vi "MonitoringProcess_DAQ.vi"(8 "error in (no error)":errorcluster, 9 "start process sync notifier":refnum<notifier>, 10 "TopLevel":refnum<class "TopLevel.lvclass">, 11 "DAQ":refnum<class "DAQ.lvclass">) -> (0 "error out":errorcluster)   [LabVIEW 2022 SP3, in "DAQ.lvclass"]
doc: "Developed by Kevin Thompson\nkevin@thompsonengineering.net\n\nCopyright 2015\nThompson Engineering, LLC"
uses:
  DAQ.lvclass
  TopLevel/TopLevel.lvclass
  MonitorProcess_DAQ SM AppData--cluster.ctl
  DataTypes/TD DAQ Settings--cluster.ctl
  DataTypes/TD DI Instrument Settings--cluster.ctl
  DataTypes/TD AI Instrument Settings--cluster.ctl
  DataTypes/TD AI InstSettings--cluster.ctl
  ProcessSupport/TD SimAI Ranges--cluster.ctl
  DAQ_Common/DataTypes/Timer_Data--Cluster.ctl
  <vilib>/TELLC/Dynamic CVT API/TD Dynamic CVT DVR--ref.ctl
  DAQ.lvclass/DAQ.ctl
  TopLevel/Typedefs/PrimingMode APIData.ctl
  TopLevel/Typedefs/PurgeMode--Enum.ctl
  TopLevel/Typedefs/PrinterHeads--Enum.ctl
  IO/Typedefs/ICP2-DO Channel Names.ctl
  DataTypes/TD DAQ Output EventSenderMode-enum.ctl
  Accessors/Get DAQ Settings.vi
  TopLevel/PurgeRequestWindow--Process.vi
  DAQ_Common/Lib/ErrorHandler/ErrorHandler.lvclass
  IO/IO.lvclass
panel:
  out "SWLED 2":bool
  out "SW LED DO":string
  out "found":bool
  out "SWLED":bool
  out "DIName":string
  in  "injected error cluster":errorcluster
  in  "inject error":bool
  in  "Stop Process":bool
  # "Simulated error injection\nfor testing and debug"
  # "This is for debugging. Process should stop from user event."
  # "Makes sure to set this value from the process caller. Using the Start asyncronous call function."
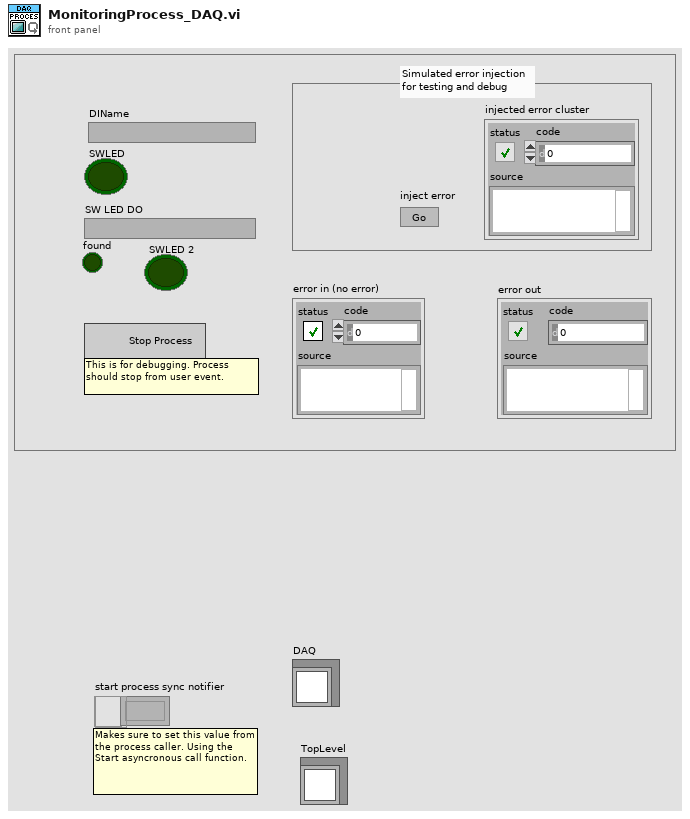
[diagram p1: front panel]
types:
  T1 = typedef "DAQ.lvclass/MonitorProcess_DAQ SM AppData--cluster.ctl" = cluster{"Core":cluster{"Current VI Ref":refnum<vi>, "process sync notifier":refnum<notifier>}, "AsyncSMQ":refnum<queue>, "DAQ Settings":T2, "SimDaqLoopIntv":i32, "ThreadSyncRndzv":T7, "vData":variant, "quitting":bool, "Self Reference":refnum<class "DAQ.lvclass">, "TopLevel":refnum<class "TopLevel.lvclass">, "Timer":T8, "DAQData Dict":T9}
  T2 = typedef "DAQ.lvclass/TD DAQ Settings--cluster.ctl" = cluster{"Simulate DAQ":bool, "DI Settings":T3[], "AI Settings":T4[], "Relay IONames":string[], "AO IONames":string[], "AO NChan SingleTask":bool}
  T3 = typedef "DAQ.lvclass/TD DI Instrument Settings--cluster.ctl" = cluster{"Disable":bool, "DI TaskName":string, "DI RefreshIntv":i32}
  T4 = typedef "DAQ.lvclass/TD AI Instrument Settings--cluster.ctl" = cluster{"Disable":bool, "AI TaskName":string, "AI InstSettings":T5, "SimAI Ranges":T6}
  T5 = typedef "DAQ.lvclass/TD AI InstSettings--cluster.ctl" = cluster{"DaqRate":dbl, "NumSamples":i32}
  T6 = typedef "DAQ.lvclass/TD SimAI Ranges--cluster.ctl" = cluster{"lo":dbl, "hi":dbl}
  T7 = typedef "Rendezvous RefNum" = refnum<k1>
  T8 = typedef "Timer_Data--Cluster.ctl" = cluster{"StartTime":timestamp, "TimerValue":dbl, "Enable":bool, "Expired":bool}
  T9 = typedef "TD Dynamic CVT DVR--ref.ctl" = refnum<data-value>
  T10 = typedef "PurgeMode--Enum.ctl" = enum16{"Pre-Purge", "Purge", "Spit", "Shake"}
  T11 = typedef "TopLevel.lvclass/PrimingMode APIData.ctl" = cluster{"Interval (s)":dbl, "PurgeDuration (s)":dbl, "Repeats":u8, "PrimingMode":T10, "Head":T12, "Frequency (Hz)":i32, "PrintWeight":dbl}
  T12 = typedef "PrinterHeads--Enum.ctl" = enum16{"-1", "1", "2", "3", "4", "5", "6"}
  T13 = typedef "DAQ.lvclass/TD DAQ Output EventSenderMode-enum.ctl" = enum16{"manual", "automation"}
  T14 = typedef "IO.lvclass/ICP2-DO Channel Names.ctl" = enum16{"None", "Meniscus Valve Open - R1", "Meniscus Valve Open - R2", "Meniscus Valve Open - R3", "Meniscus Valve Open - R4", "Meniscus Valve Open - R5", "Meniscus Valve Open - R6", "Ink Flow Valve Open - R1", "Ink Flow Valve Open - R2", "Ink Flow Valve Open - R3", "Ink Flow Valve Open - R4", "Ink Flow Valve Open - R5", "Ink Flow Valve Open - R6", "SW_LED - Ink Valve - R1", "SW_LED - Ink Valve - R2", "SW_LED - Ink Valve - R3", "Recirc Pump On - R1", "Recirc Pump On - R2", "Recirc Pump On - R3", "Recirc Pump On - R4", "Recirc Pump On - R5", "Recirc Pump On - R6", "SW_LED - Ink Valve - R4", "SW_LED - Ink Valve - R5", "SW_LED - Ink Valve - R6"}
  T15 = enum32{"Invalid", "Standard", "Closed", "Hidden", "Minimized", "Maximized"}
  T16 = cluster{"Prime 1":string, "Prime 2":string, "Prime 3":string, "Prime 4":string, "Prime 5":string, "Prime 6":string}
  T17 = typedef "processMode--enum.ctl" = enum16{"Short Idle", "Long Idle ", "C30_Process", "S30_Process"}
  T18 = typedef "ProcessMode--Cluster.ctl" = cluster{"Head Array":u8[], "Head Enable":bool[], "HeadTemp[]":dbl[], "MeniscusPress[]":dbl[], "Recirc[]":bool[], "ProcessModeEnum":T17, "ProcessModeStr":string, "ColorPlane[]":string[]}
  T19 = typedef "TopLevel.lvclass/UserEvents.ctl" = cluster{"API Incoming Event":refnum<user-event>, "API Executed Event":refnum<user-event>, "API Return Event":refnum<user-event>, "Exit Event":refnum<user-event>, "StatusChanged":refnum<user-event>, "DLP GUI Config Changed":refnum<user-event>, "AppEvent":refnum<user-event>, "Login Event":refnum<user-event>, "HeadPrimeStatusEvent":refnum<user-event>}
  T20 = typedef "DAQ.lvclass/TD PublicEvents--cluster.ctl" = cluster{"DaqOutputCmd Ev":refnum<user-event>, "stop process":refnum<user-event>, "DAQ.AsyncCmd Event":refnum<user-event>, "DAQStateChanged Event":refnum<user-event>, "DAQ.AsyncMsg Event":refnum<user-event>, "DAQ_DO_StatusEvent":refnum<user-event>, "DIStateChangeEv":refnum<user-event>, "UI StateChanged":refnum<user-event>, "PurgeTimerEvent":refnum<user-event>}
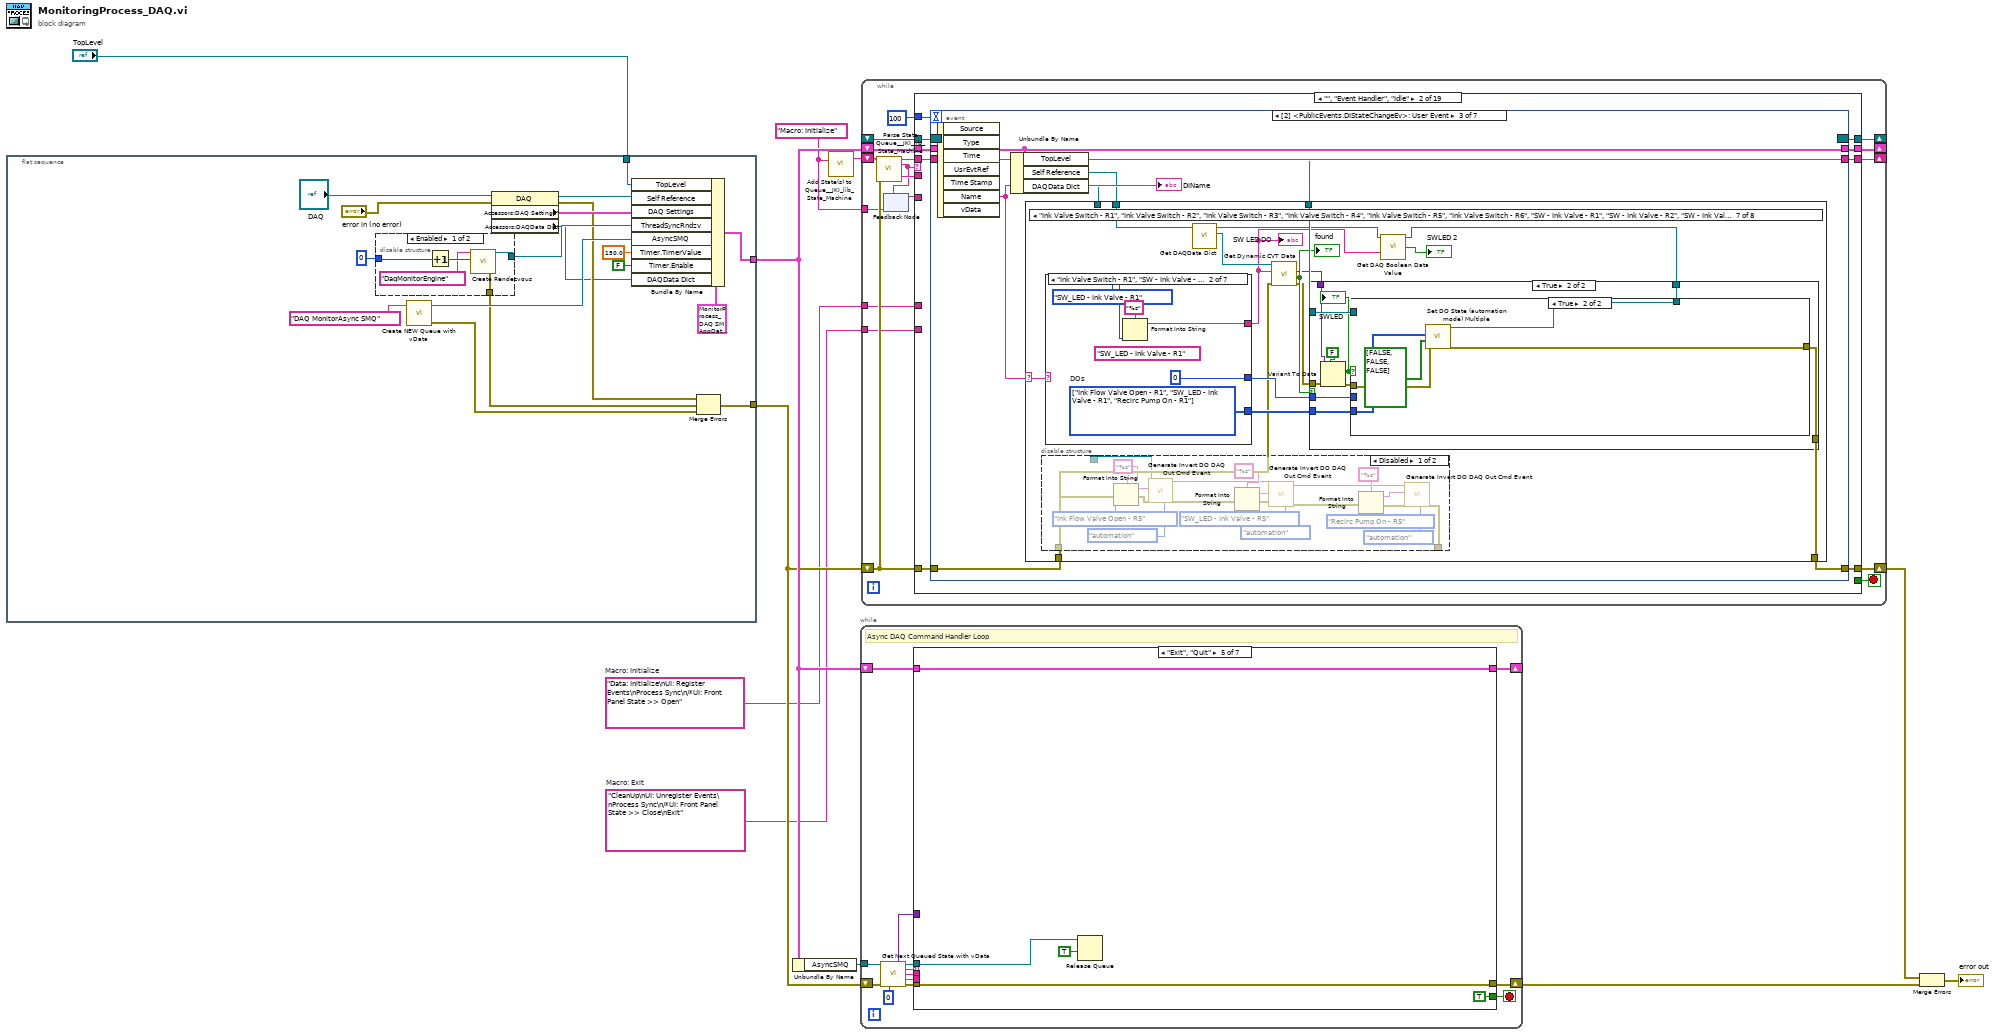
[diagram p0: block diagram]
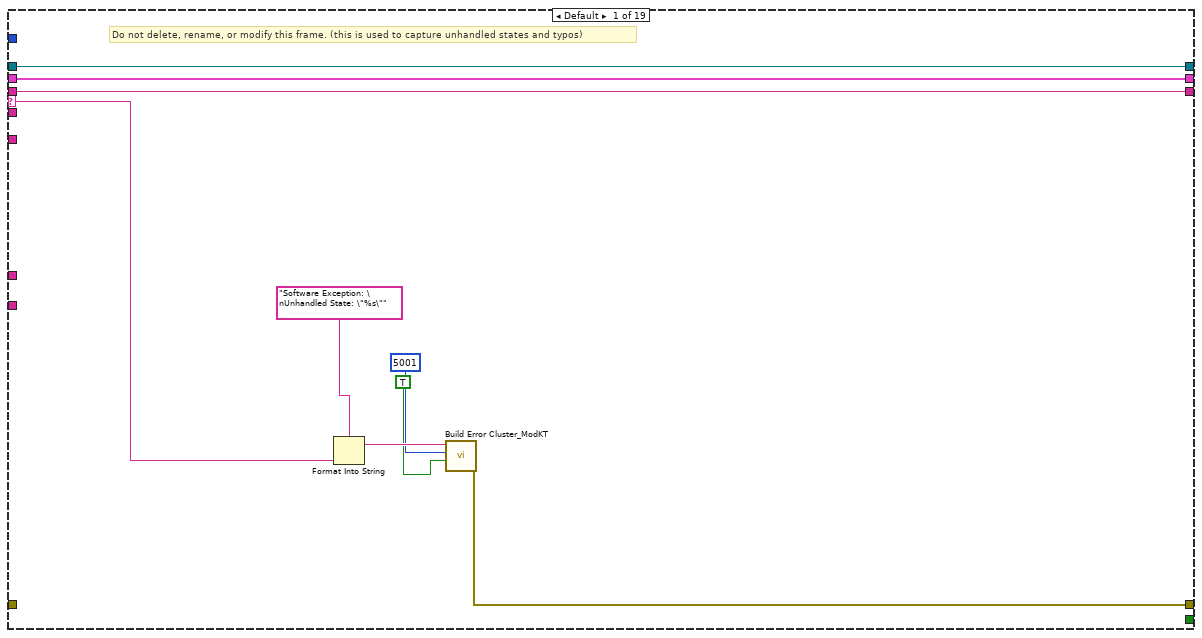
[diagram p2: hidden frame]
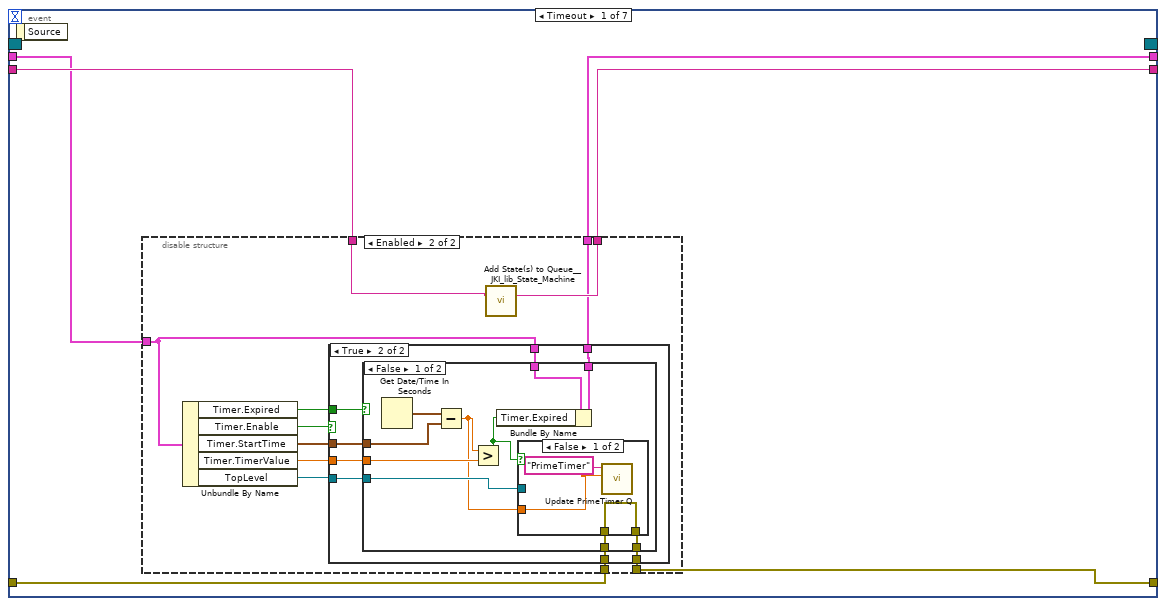
[diagram p3: hidden frame]
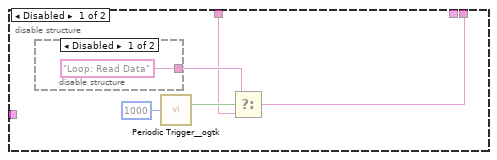
[diagram p4: hidden frame]
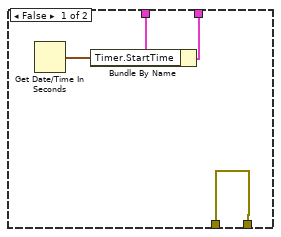
[diagram p6: hidden frame]
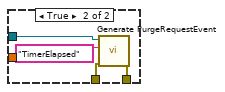
[diagram p7: hidden frame]
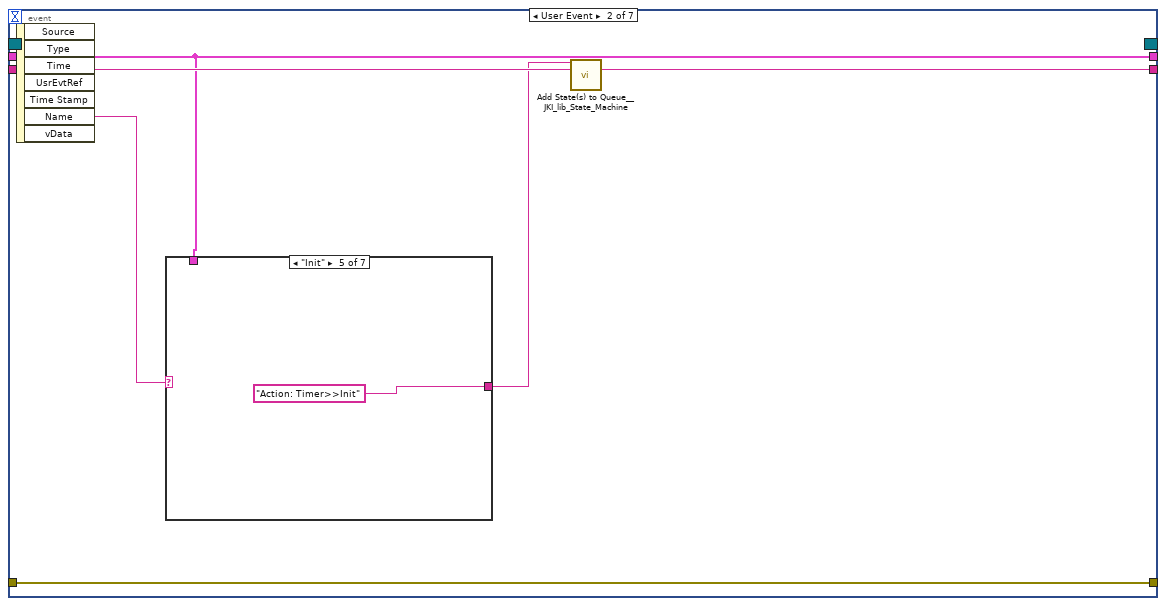
[diagram p9: hidden frame]
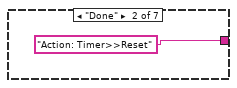
[diagram p11: hidden frame]
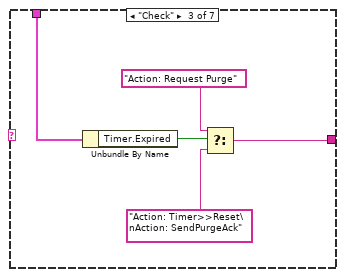
[diagram p12: hidden frame]
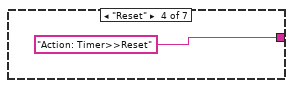
[diagram p13: hidden frame]
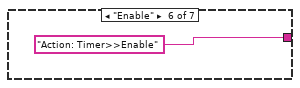
[diagram p14: hidden frame]
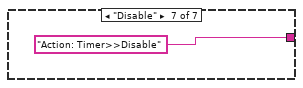
[diagram p15: hidden frame]
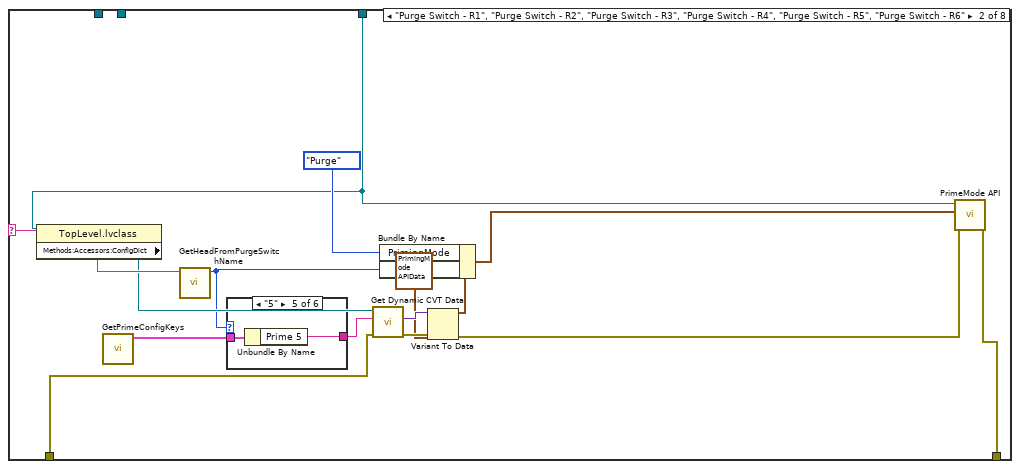
[diagram p17: hidden frame]
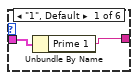
[diagram p18: hidden frame]
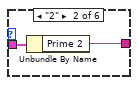
[diagram p19: hidden frame]
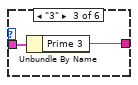
[diagram p20: hidden frame]
diagram:
  w4 = "Data: Initialize\nUI: Register Events\nProcess Sync\n/*UI: Front Panel State >> Open"  # Macro: Initialize
  w3 = "CleanUp\nUI: Unregister Events\nProcess Sync\n/*UI: Front Panel State >> Close\nExit"  # Macro: Exit
  w2 = "Macro: Initialize"
  n1 = flat-sequence {
    tunnel: [w29] -> w9
    tunnel: [w23] -> w8
    tunnel: "TopLevel" -> [w15]
    frame #0 {
      n2 = disable-structure shown="Enabled" {
        disable-tunnel: [w34 _] -> w25
        disable-tunnel: [w33 _] -> w24
        disable-tunnel: 0 -> [w30 _]
        frame Enabled {
          n3 = Increment(x=w30) -> (x+1=w32:i32)
          n4 = call <vilib>:"Create Rendezvous.vi"("size (2)"=w32, "name (unnamed)"="DaqMonitorEngine" ("ProcVI ID")) -> ("error out"=w33:errorcluster, "rendezvous"=w34:T7)  [unwired: 3 in, 1 out]
        }
        frame Disabled {
        }
      }
      n5 = call <vilib>:"Create NEW Queue with vData.vi"("Name (SMQ)"="DAQ MonitorAsync SMQ") -> ("error out"=w27:errorcluster, "queue out"=w26:refnum<queue>)  [unwired: 3 in]
      n6 = property class="DAQ"(reference="DAQ", error in="error in (no error)") -> (reference out=w20:refnum<class "DAQ.lvclass">, error out=w18:errorcluster, "Accessors:DAQ Settings*"=w21:T2, "Accessors:DAQData Dict"=w12:T9)
      n7 = Bundle By Name(cluster=T1 {"Core"={"Current VI Ref"=refnum, "process sync notifier"=refnum}, "AsyncSMQ"=refnum, "DAQ Settings"={"Simulate DAQ"=FALSE, "DI Settings"=[], "AI Settings"=[], "Relay IONames"=[], "AO IONames"=[], "AO NChan SingleTask"=FALSE}, "SimDaqLoopIntv"=0, "ThreadSyncRndzv"=refnum, "vData"=variant, "quitting"=FALSE, "Self Reference"=refnum, "TopLevel"=refnum, "Timer"={"StartTime"=timestamp(0 s since 1904-01-01), "TimerValue"=0.0, "Enable"=FALSE, "Expired"=FALSE}, "DAQData Dict"=refnum} ("DAQ Process AppData"), "TopLevel"=w15, "Self Reference"=w20, "DAQ Settings"=w21, "ThreadSyncRndzv"=w25, "AsyncSMQ"=w26, "Timer.TimerValue"=150.0, "Timer.Enable"=FALSE, "DAQData Dict"=w12) -> (w29:T1)
      n8 = Merge Errors(w18, w24, w27) -> (w23:errorcluster)
    }
  }
  n9 = Unbundle By Name(w9) -> ("AsyncSMQ"=w10:refnum<queue>)
  n10 = call <vilib>:"Add State(s) to Queue__JKI_lib_State_Machine.vi"("State(s) in (\"\")"=w2) -> ("States Out"=w11:string)  [unwired: 14 in]
  n11 = while {
    shift-right: [w36] -> _
    shift-left: w9 -> [w37]
    tunnel: w10 -> [w47]
    shift-right: [w39] -> w7
    shift-left: w8 -> [w41]
    stop <- w38 stop-if-true
    # "Async DAQ Command Handler Loop"
    n12 = call <vilib>:"Get Next Queued State with vData.vi"("queue in"=w47, "error in (no error)"=w41, "timeout (100)"=0) -> ("vData out"=w42:variant, "queue out"=w45:refnum<queue>, "Next State"=w46:string, "queued msg"=w44:string, "Prev State"=w43:string, "error out"=w40:errorcluster)  [unwired: 6 in, 1 out]
    n13 = case shown="\"Exit\", \"Quit\"" w46 {
      tunnel: w40 -> [_ w57 w67 _ w75 w82 w85]
      tunnel: w45 -> [_ _ _ w71 w76 _ _]
      tunnel: w44 -> [_ _ _ _ _ _ _]
      selector: w46 -> [w48 _ _ _ _ _ _]
      tunnel: w43 -> [_ w56 _ _ _ _ _]
      tunnel: w42 -> [_ _ _ _ _ _ _]
      tunnel: [w49 w55 w67 w73 w75 w81 w85] -> w39
      tunnel: [_ _ _ _ TRUE _ _] -> w38
      tunnel: w37 -> [w54 w58 w66 w74 w78 w83 w84]
      tunnel: [w54 w58 w66 w74 w78 w83 w84] -> w36
      frame Default {
        n14 = Format Into String(format string="Software Exception: \nUnhandled State: \"%s\"", w48) -> (resulting string=w51:string)  [unwired: 2 in, 1 out]
        n15 = call <vilib>:"Build Error Cluster_ModKT .vi"("Prepend String (\"\")"=w51, "code"=5001, "error? (F)"=TRUE ("error?")) -> ("error out"=w49:errorcluster)  [unwired: 4 in, 1 out]
      }
      frame "Error Handler" {
        n16 = disable-structure shown="Enabled" {
          disable-tunnel: w57 -> [w61 w65]
          disable-tunnel: w56 -> [w60 _]
          disable-tunnel: [w59 errorcluster {"status"=FALSE, "code"=0, "source"=""} ("error constant")] -> w55
          frame Enabled {
            n17 = Concatenate Strings("Previous State: ", w60) -> (w63:string)
            n18 = call "Handle Error SM.vi"("error in (no error)"=w61, "CustomMessage"=w63) -> ("error out"=w59:errorcluster)  [unwired: 7 in, 2 out]
          }
          frame Disabled {
            n19 = call <vilib>:"General Error Handler.vi"("error in (no error)"=w65) -> ()  [unwired: 10 in, 5 out]
          }
        }
      }
      frame "Initialize" {
      }
      frame "CleanUp", "Macro: Exit" {
        # "Do any necessary async loop clean up here before quitting"
        n20 = Flush Queue(queue=w71, error in (no error)=errorcluster {"status"=FALSE, "code"=0, "source"=""}) -> (queue out=w72:refnum<queue>, error out=w70:errorcluster)  [unwired: 1 out]
        n21 = call <vilib>:"Add State to Queue with vData.vi"("queue in"=w72, "state in"="Exit", "error in"=w70) -> ("error out"=w73:errorcluster)  [unwired: 9 in, 3 out]
      }
      frame "Exit", "Quit" {
        n22 = Release Queue(queue=w76, force destroy? (F)=TRUE) -> ()  [unwired: 1 in, 3 out]
      }
      frame "", "Idle" {
        n23 = call <userlib>:"Wait (ms)__ogtk.vi"("error in (no error)"=w82, "milliseconds to wait"=u32 100) -> ("error out"=w81:errorcluster)  [unwired: 8 in, 1 out]
      }
      frame "------ Cmd ------" {
      }
    }
  }
  n24 = while {
    shift-right: [w96] -> _
    shift-left: w9 -> [w95]
    shift-right: [w99] -> w6
    shift-left: w8 -> [w94]
    shift-right: [w98] -> _
    shift-left: w11 -> [w100]
    shift-right: [w92] -> _
    shift-left: _ -> [w93]
    tunnel: w4 -> [w90]
    tunnel: w3 -> [w89]
    tunnel: w2 -> [w87]
    stop <- w97 stop-if-true
    n25 = call <vilib>:"Parse State Queue__JKI_lib_State_Machine.vi"("State Queue"=w100, "Error In (no error)"=w94) -> ("Remaining States"=w102:string, "Current State"=w88:string, "Arguments"=w101:string)  [unwired: 11 in]
    n26 = feedback #1(w87) -> (w86:string)
    n27 = feedback-in #1(w88) -> ()
    n28 = case shown="\"\", \"Event Handler\", \"Idle\"" w88 {
      selector: w88 -> [w103 _ _ _ _ _ _ _ _ _ _ _ _ _ _ _ _ _ _]
      tunnel: w102 -> [w110 w120 w459 w476 w485 w493 w499 w509 w512 w519 w530 w533 w541 w575 w580 w583 w591 w609 w614]
      tunnel: w101 -> [_ _ _ _ _ _ _ _ _ _ _ _ w535 _ _ _ _ _ w612]
      tunnel: w95 -> [w111 w118 w457 w471 w486 w491 w498 w502 w511 w516 w523 w532 w538 w573 w579 w582 w589 w607 w610]
      tunnel: [w104 w117 w448 w470 w487 w495 w500 w503 w513 w517 w521 w534 w537 w572 w576 w584 w586 w594 w615] -> w99
      tunnel: w94 -> [_ w116 w455 w473 w488 w495 w500 w503 w513 w517 w520 w534 w536 w565 w576 w584 w585 w596 w615]
      tunnel: [w110 w119 w459 w475 w485 w493 w499 w509 w512 w518 w529 w533 w541 w575 w580 w583 w591 w609 w614] -> w98
      tunnel: [_ _ _ _ _ TRUE _ _ _ _ _ _ _ _ _ _ _ _ _] -> w97
      tunnel: [w111 w115 w457 w471 w486 w491 w498 w505 w511 w516 w527 w532 w538 w573 w579 w582 w589 w593 w611] -> w96
      tunnel: w93 -> [w109 w114 w458 w474 w484 w492 w497 w508 w510 w515 w528 w531 w540 _ w577 w581 w590 w608 w613]
      tunnel: [w109 w113 w458 w474 w484 w492 w497 w508 w510 w515 w528 w531 w540 w574 w577 w581 w590 w608 w613] -> w92
      tunnel: 100 ("Timeout") -> [_ w112 _ _ _ _ _ _ _ _ _ _ _ _ _ _ _ _ _]
      tunnel: w86 -> [_ _ _ w472 _ _ _ _ _ _ _ _ _ _ _ _ _ _ _]
      tunnel: w90 -> [_ _ _ _ _ _ _ _ _ w514 _ _ _ _ _ _ _ _ _]
      tunnel: w89 -> [_ _ _ _ _ _ _ _ _ _ w525 _ _ _ _ _ _ _ _]
      frame Default {
        # "Do not delete, rename, or modify this frame. (this is used to capture unhandled states and typos)"
        n29 = Format Into String(format string="Software Exception: \nUnhandled State: \"%s\"", w103) -> (resulting string=w107:string)  [unwired: 2 in, 1 out]
        n30 = call <vilib>:"Build Error Cluster_ModKT .vi"("Prepend String (\"\")"=w107, "code"=5001, "error? (F)"=TRUE ("error?")) -> ("error out"=w104:errorcluster)  [unwired: 4 in, 1 out]
      }
      frame "", "Event Handler", "Idle" {
        n31 = event "executes when the state queue is empty" shown="[2] <PublicEvents.DIStateChangeEv>: User Event" {
          selector: w114 -> [_ _ _ _ _ _ _]
          dyn-events: [_ _ _ _ _ _ _] -> w113
          timeout: w112 -> [_ _ _ _ _ _ _]
          tunnel: w120 -> [w126 w178 w198 w431 _ w440 w447]
          tunnel: [w125 w179 w198 w432 w436 w442 w447] -> w119
          tunnel: w118 -> [w123 w175 w194 w433 w438 w443 w446]
          tunnel: [w122 w180 w196 w434 w439 w444 "injected error cluster"] -> w117
          tunnel: w116 -> [w121 w180 w195 w434 w439 w444 _]
          tunnel: [w124 w175 w194 w433 w437 w443 w446] -> w115
          event Timeout {
            n32 = event-data() -> ()  [unwired: 1 in, 1 out]
            n33 = disable-structure shown="Enabled" {
              disable-tunnel: w126 -> [w128 w140]
              disable-tunnel: [w127 w141] -> w125
              disable-tunnel: w123 -> [_ w138]
              disable-tunnel: [_ w137] -> w124
              disable-tunnel: w121 -> [_ w134]
              disable-tunnel: [_ w133] -> w122
              frame Disabled {
                n34 = disable-structure shown="Disabled" {
                  disable-tunnel: ["Loop: Read Data" _] -> w129
                  frame Disabled {
                  }
                  frame Enabled {
                  }
                }
                n35 = call <userlib>:"Periodic Trigger__ogtk.vi"("time (ms)"=u32 1000) -> ("Triggered"=w130:bool)  [unwired: 12 in, 2 out]
                n36 = Select(t=w129, s=w130, f=w128) -> (s? t:f=w127:string)
              }
              frame Enabled {
                n37 = Unbundle By Name(w138) -> ("Timer.Expired"=w136:bool, "Timer.Enable"=w139:bool, "Timer.StartTime"=w143:timestamp, "Timer.TimerValue"=w142:dbl, "TopLevel"=w135:refnum<class "TopLevel.lvclass">)
                n38 = case shown="True" w139 {
                  tunnel: w143 -> [_ w155]
                  tunnel: w142 -> [_ w154]
                  tunnel: w138 -> [w147 w153]
                  tunnel: [w145 w152] -> w137
                  tunnel: w136 -> [_ w151]
                  tunnel: w135 -> [_ w150]
                  tunnel: w134 -> [w144 w149]
                  tunnel: [w144 w148] -> w133
                  frame False {
                    n39 = Get Date/Time In Seconds() -> (seconds since 1Jan1904=w146:timestamp)
                    n40 = Bundle By Name(cluster=w147, "Timer.StartTime"=w146) -> (w145:T1)
                  }
                  frame True {
                    n41 = case shown="False" w151 {
                      tunnel: w155 -> [w164 _]
                      tunnel: w154 -> [w163 _]
                      tunnel: w153 -> [w162 w174]
                      tunnel: [w161 w174] -> w152
                      tunnel: w150 -> [w159 _]
                      tunnel: w149 -> [w158 w173]
                      tunnel: [w157 w173] -> w148
                      frame False {
                        n42 = Get Date/Time In Seconds() -> (seconds since 1Jan1904=w165:timestamp)
                        n43 = Subtract(x=w165, y=w164) -> (x-y=w156:dbl)
                        n44 = Greater?(x=w156, y=w163) -> (0:w160:bool)
                        n45 = Bundle By Name(cluster=w162, "Timer.Expired"=w160) -> (w161:T1)
                        n46 = case shown="False" w160 {
                          tunnel: w159 -> [_ w171]
                          tunnel: w158 -> [w168 w170]
                          tunnel: [w168 w169] -> w157
                          tunnel: w156 -> [w167 _]
                          frame False {
                            n47 = call "Update PrimeTimer Q.vi"("elapsed time (s)"=w167, "PrimeTimerName"="PrimeTimer") -> ()  [unwired: 6 in]
                          }
                          frame True {
                            n48 = call-dynamic "Generate PurgeRequestEvent.vi"("error in (no error)"=w170, "Command"="TimerElapsed", "TopLevel in"=w171) -> ("error out"=w169:errorcluster)  [unwired: 7 in, 1 out]
                          }
                        }
                      }
                      frame True {
                      }
                    }
                  }
                }
                n49 = call <vilib>:"Add State(s) to Queue__JKI_lib_State_Machine.vi"("State(s) in (\"\")"=w140) -> ("States Out"=w141:string)  [unwired: 14 in]
              }
            }
          }
          event User Event {
            n50 = event-data() -> ("Name"=w176:string)  [unwired: 1 in, 6 out]
            n51 = case shown="\"Init\"" w176 {
              tunnel: [_ "Action: Timer>>Reset" ("State(s) in Front (\"\")") w182 "Action: Timer>>Reset" ("State(s) in Front (\"\")") "Action: Timer>>Init" ("State(s) in Front (\"\")") "Action: Timer>>Enable" ("State(s) in Front (\"\")") "Action: Timer>>Disable" ("State(s) in Front (\"\")")] -> w177
              tunnel: w175 -> [_ _ w186 _ _ _ _]
              frame "False", Default {
              }
              frame "Done" {
              }
              frame "Check" {
                n52 = Unbundle By Name(w186) -> ("Timer.Expired"=w185:bool)
                n53 = Select(t="Action: Request Purge", s=w185, f="Action: Timer>>Reset\nAction: SendPurgeAck") -> (s? t:f=w182:string)
              }
              frame "Reset" {
              }
              frame "Init" {
              }
              frame "Enable" {
              }
              frame "Disable" {
              }
            }
            n54 = call <vilib>:"Add State(s) to Queue__JKI_lib_State_Machine.vi"("State(s) in Front (\"\")"=w177, "State(s) in (\"\")"=w178) -> ("States Out"=w179:string)  [unwired: 13 in]
          }
          event User Event {
            n55 = event-data() -> ("Name"=w197:string)  [unwired: 1 in, 6 out]
            "DIName" <- w197
            n56 = Unbundle By Name(w194) -> ("TopLevel"=w192:refnum<class "TopLevel.lvclass">, "Self Reference"=w193:refnum<class "DAQ.lvclass">, "DAQData Dict"=w191:T9)
            n57 = case shown="\"Ink Valve Switch - R1\", \"Ink Valve Switch - R2\", \"Ink Valve Switch - R3\", \"Ink Valve Switch - R4\", \"Ink Valve Switch - R5\", \"Ink Valve Switch - R6\", \"SW - Ink Valve - R1\", \"SW - Ink Valve - R2\", \"SW - Ink Valve - R3\", \"SW - Ink Valve - R4\", \"SW - Ink Valve - R5\", \"SW - Ink Valve - R6\"" w197 {
              selector: w197 -> [_ w213 _ _ _ _ w325 _]
              tunnel: w193 -> [_ _ w245 w267 w289 w311 w319 w426]
              tunnel: w195 -> [w199 w200 w238 w260 w282 w304 w324 w419]
              tunnel: [w199 w214 w229 w250 w272 w294 w327 w409] -> w196
              tunnel: w192 -> [_ w210 _ _ _ _ w328 _]
              tunnel: w191 -> [_ _ _ _ _ _ _ _]
              frame "False", Default {
              }
              frame "Purge Switch - R1", "Purge Switch - R2", "Purge Switch - R3", "Purge Switch - R4", "Purge Switch - R5", "Purge Switch - R6" {
                n58 = property class="TopLevel.lvclass"(reference=w210) -> ("Methods:Accessors:ConfigDict"=w209:T9)  [unwired: 1 in, 2 out]
                n59 = call "GetPrimeConfigKeys.vi"() -> ("Prime Names"=w207:T16)  [unwired: 11 in]
                n60 = call "GetHeadFromPurgeSwitchName.vi"("input string"=w213) -> ("output 1"=w208:T12)  [unwired: 9 in, 1 out]
                n61 = case shown="\"5\"" w208 {
                  tunnel: w207 -> [w216 w218 w220 w222 w224 w226]
                  tunnel: [w215 w217 w219 w221 w223 w225] -> w206
                  frame "1", Default {
                    n62 = Unbundle By Name(w216) -> ("Prime 1"=w215:string)
                  }
                  frame "2" {
                    n63 = Unbundle By Name(w218) -> ("Prime 2"=w217:string)
                  }
                  frame "3" {
                    n64 = Unbundle By Name(w220) -> ("Prime 3"=w219:string)
                  }
                  frame "4" {
                    n65 = Unbundle By Name(w222) -> ("Prime 4"=w221:string)
                  }
                  frame "5" {
                    n66 = Unbundle By Name(w224) -> ("Prime 5"=w223:string)
                  }
                  frame "6" {
                    n67 = Unbundle By Name(w226) -> ("Prime 6"=w225:string)
                  }
                }
                n68 = call <vilib>:"Get Dynamic CVT Data.vi"("error in (no error)"=w200, "DataName"=w206, "dCVT DVR"=w209) -> ("error out"=w205:errorcluster, "value"=w204:variant)  [unwired: 5 in, 2 out]
                n69 = Variant To Data(error in=w205, type=T11 {"Interval (s)"=0.1, "PurgeDuration (s)"=0.1, "Repeats"=0, "PrimingMode"=enum."Purge", "Head"=enum."1", "Frequency (Hz)"=0, "PrintWeight"=0.1} ("Pre Purge API Data"), Variant=w204) -> (data=w202:T11, error out=w201:errorcluster)
                n70 = Bundle By Name(cluster=w202, "PrimingMode"=PurgeMode--Enum."Purge", "Head"=w208) -> (w211:T11)
                n71 = call-dynamic "PrimeMode API.vi"("error in (no error)"=w201, "Pre Purge API Data"=w211, "TopLevel in"=w210) -> ("error out"=w214:errorcluster)  [unwired: 7 in, 1 out]
              }
              frame "old LED1" {
                n72 = Format Into String(format string="%s", error in=w238, ICP2-DO_Channel_Names."Ink Flow Valve Open - R1" ("DO Channel")) -> (resulting string=w246:string, error out=w241:errorcluster)  [unwired: 1 in]
                n73 = call "Generate Invert DO DAQ Out Cmd Event.vi"("mode (manual)"=TD_DAQ_Output_EventSenderMode-enum."automation", "error in (no error)"=w241, "DO IOName"=w246, "DAQ"=w245) -> ("error out"=w240:errorcluster, "DAQ"=w242:refnum<class "DAQ.lvclass">)  [unwired: 6 in]
                n74 = Format Into String(format string="%s", error in=w240, ICP2-DO_Channel_Names."SW_LED - Ink Valve - R1" ("DO Channel")) -> (resulting string=w237:string, error out=w239:errorcluster)  [unwired: 1 in]
                n75 = call "Generate Invert DO DAQ Out Cmd Event.vi"("mode (manual)"=TD_DAQ_Output_EventSenderMode-enum."automation", "error in (no error)"=w239, "DO IOName"=w237, "DAQ"=w242) -> ("error out"=w228:errorcluster, "DAQ"=w230:refnum<class "DAQ.lvclass">)  [unwired: 6 in]
                n76 = Format Into String(format string="%s", error in=w228, ICP2-DO_Channel_Names."Recirc Pump On - R1" ("DO Channel")) -> (resulting string=w231:string, error out=w227:errorcluster)  [unwired: 1 in]
                n77 = call "Generate Invert DO DAQ Out Cmd Event.vi"("mode (manual)"=TD_DAQ_Output_EventSenderMode-enum."automation", "error in (no error)"=w227, "DO IOName"=w231, "DAQ"=w230) -> ("error out"=w229:errorcluster)  [unwired: 6 in, 1 out]
              }
              frame "old LED2" {
                n78 = Format Into String(format string="%s", error in=w260, ICP2-DO_Channel_Names."Ink Flow Valve Open - R2" ("DO Channel")) -> (resulting string=w268:string, error out=w263:errorcluster)  [unwired: 1 in]
                n79 = call "Generate Invert DO DAQ Out Cmd Event.vi"("mode (manual)"=TD_DAQ_Output_EventSenderMode-enum."automation", "error in (no error)"=w263, "DO IOName"=w268, "DAQ"=w267) -> ("error out"=w262:errorcluster, "DAQ"=w264:refnum<class "DAQ.lvclass">)  [unwired: 6 in]
                n80 = Format Into String(format string="%s", error in=w262, ICP2-DO_Channel_Names."SW_LED - Ink Valve - R2" ("DO Channel")) -> (resulting string=w259:string, error out=w261:errorcluster)  [unwired: 1 in]
                n81 = call "Generate Invert DO DAQ Out Cmd Event.vi"("mode (manual)"=TD_DAQ_Output_EventSenderMode-enum."automation", "error in (no error)"=w261, "DO IOName"=w259, "DAQ"=w264) -> ("error out"=w251:errorcluster, "DAQ"=w252:refnum<class "DAQ.lvclass">)  [unwired: 6 in]
                n82 = Format Into String(format string="%s", error in=w251, ICP2-DO_Channel_Names."Recirc Pump On - R2" ("DO Channel")) -> (resulting string=w254:string, error out=w253:errorcluster)  [unwired: 1 in]
                n83 = call "Generate Invert DO DAQ Out Cmd Event.vi"("mode (manual)"=TD_DAQ_Output_EventSenderMode-enum."automation", "error in (no error)"=w253, "DO IOName"=w254, "DAQ"=w252) -> ("error out"=w250:errorcluster)  [unwired: 6 in, 1 out]
              }
              frame "old LED3" {
                n84 = Format Into String(format string="%s", error in=w282, ICP2-DO_Channel_Names."Ink Flow Valve Open - R3" ("DO Channel")) -> (resulting string=w290:string, error out=w285:errorcluster)  [unwired: 1 in]
                n85 = call "Generate Invert DO DAQ Out Cmd Event.vi"("mode (manual)"=TD_DAQ_Output_EventSenderMode-enum."automation", "error in (no error)"=w285, "DO IOName"=w290, "DAQ"=w289) -> ("error out"=w284:errorcluster, "DAQ"=w286:refnum<class "DAQ.lvclass">)  [unwired: 6 in]
                n86 = Format Into String(format string="%s", error in=w284, ICP2-DO_Channel_Names."SW_LED - Ink Valve - R3" ("DO Channel")) -> (resulting string=w281:string, error out=w283:errorcluster)  [unwired: 1 in]
                n87 = call "Generate Invert DO DAQ Out Cmd Event.vi"("mode (manual)"=TD_DAQ_Output_EventSenderMode-enum."automation", "error in (no error)"=w283, "DO IOName"=w281, "DAQ"=w286) -> ("error out"=w273:errorcluster, "DAQ"=w274:refnum<class "DAQ.lvclass">)  [unwired: 6 in]
                n88 = Format Into String(format string="%s", error in=w273, ICP2-DO_Channel_Names."Recirc Pump On - R3" ("DO Channel")) -> (resulting string=w276:string, error out=w275:errorcluster)  [unwired: 1 in]
                n89 = call "Generate Invert DO DAQ Out Cmd Event.vi"("mode (manual)"=TD_DAQ_Output_EventSenderMode-enum."automation", "error in (no error)"=w275, "DO IOName"=w276, "DAQ"=w274) -> ("error out"=w272:errorcluster)  [unwired: 6 in, 1 out]
              }
              frame "old LED4" {
                n90 = Format Into String(format string="%s", error in=w304, ICP2-DO_Channel_Names."Ink Flow Valve Open - R4" ("DO Channel")) -> (resulting string=w312:string, error out=w307:errorcluster)  [unwired: 1 in]
                n91 = call "Generate Invert DO DAQ Out Cmd Event.vi"("mode (manual)"=TD_DAQ_Output_EventSenderMode-enum."automation", "error in (no error)"=w307, "DO IOName"=w312, "DAQ"=w311) -> ("error out"=w306:errorcluster, "DAQ"=w308:refnum<class "DAQ.lvclass">)  [unwired: 6 in]
                n92 = Format Into String(format string="%s", error in=w306, ICP2-DO_Channel_Names."SW_LED - Ink Valve - R4" ("DO Channel")) -> (resulting string=w303:string, error out=w305:errorcluster)  [unwired: 1 in]
                n93 = call "Generate Invert DO DAQ Out Cmd Event.vi"("mode (manual)"=TD_DAQ_Output_EventSenderMode-enum."automation", "error in (no error)"=w305, "DO IOName"=w303, "DAQ"=w308) -> ("error out"=w295:errorcluster, "DAQ"=w296:refnum<class "DAQ.lvclass">)  [unwired: 6 in]
                n94 = Format Into String(format string="%s", error in=w295, ICP2-DO_Channel_Names."Recirc Pump On - R4" ("DO Channel")) -> (resulting string=w298:string, error out=w297:errorcluster)  [unwired: 1 in]
                n95 = call "Generate Invert DO DAQ Out Cmd Event.vi"("mode (manual)"=TD_DAQ_Output_EventSenderMode-enum."automation", "error in (no error)"=w297, "DO IOName"=w298, "DAQ"=w296) -> ("error out"=w294:errorcluster)  [unwired: 6 in, 1 out]
              }
              frame "Ink Valve Switch - R1", "Ink Valve Switch - R2", "Ink Valve Switch - R3", "Ink Valve Switch - R4", "Ink Valve Switch - R5", "Ink Valve Switch - R6", "SW - Ink Valve - R1", "SW - Ink Valve - R2", "SW - Ink Valve - R3", "SW - Ink Valve - R4", "SW - Ink Valve - R5", "SW - Ink Valve - R6" {
                n96 = disable-structure shown="Disabled" {
                  disable-tunnel: w324 -> [w398 _]
                  disable-tunnel: [w388 _] -> _
                  disable-tunnel: _ -> [w386 _]
                  frame Disabled {
                    n97 = Format Into String(format string="%s", error in=w398, ICP2-DO_Channel_Names."Ink Flow Valve Open - R5" ("DO Channel")) -> (resulting string=w405:string, error out=w401:errorcluster)  [unwired: 1 in]
                    n98 = call "Generate Invert DO DAQ Out Cmd Event.vi"("mode (manual)"=TD_DAQ_Output_EventSenderMode-enum."automation", "error in (no error)"=w401, "DO IOName"=w405, "DAQ"=w386) -> ("error out"=w400:errorcluster, "DAQ"=w402:refnum<class "DAQ.lvclass">)  [unwired: 6 in]
                    n99 = Format Into String(format string="%s", error in=w400, ICP2-DO_Channel_Names."SW_LED - Ink Valve - R5" ("DO Channel")) -> (resulting string=w397:string, error out=w399:errorcluster)  [unwired: 1 in]
                    n100 = call "Generate Invert DO DAQ Out Cmd Event.vi"("mode (manual)"=TD_DAQ_Output_EventSenderMode-enum."automation", "error in (no error)"=w399, "DO IOName"=w397, "DAQ"=w402) -> ("error out"=w389:errorcluster, "DAQ"=w390:refnum<class "DAQ.lvclass">)  [unwired: 6 in]
                    n101 = Format Into String(format string="%s", error in=w389, ICP2-DO_Channel_Names."Recirc Pump On - R5" ("DO Channel")) -> (resulting string=w392:string, error out=w391:errorcluster)  [unwired: 1 in]
                    n102 = call "Generate Invert DO DAQ Out Cmd Event.vi"("mode (manual)"=TD_DAQ_Output_EventSenderMode-enum."automation", "error in (no error)"=w391, "DO IOName"=w392, "DAQ"=w390) -> ("error out"=w388:errorcluster)  [unwired: 6 in, 1 out]
                  }
                  frame Enabled {
                  }
                }
                n103 = case shown="\"Ink Valve Switch - R1\", \"SW - Ink Valve - R1\"" w325 {
                  tunnel: [_ w366 "SW_LED - Ink Valve - R2" "SW_LED - Ink Valve - R3" "SW_LED - Ink Valve - R4" "SW_LED - Ink Valve - R5" "SW_LED - Ink Valve - R6"] -> w316
                  tunnel: [w364 w370 w373 w376 w379 w382 w385] -> w329
                  tunnel: [0 ("index") 0 ("index") 1 ("index") 2 ("index") 3 ("index") 4 ("index") 5 ("index")] -> w326
                  frame Default {
                    w364 = T14[] [] items=["None", "Meniscus Valve Open - R1", "Meniscus Valve Open - R2", "Meniscus Valve Open - R3", "Meniscus Valve Open - R4", "Meniscus Valve Open - R5", "Meniscus Valve Open - R6", "Ink Flow Valve Open - R1", "Ink Flow Valve Open - R2", "Ink Flow Valve Open - R3", "Ink Flow Valve Open - R4", "Ink Flow Valve Open - R5", "Ink Flow Valve Open - R6", "SW_LED - Ink Valve - R1", "SW_LED - Ink Valve - R2", "SW_LED - Ink Valve - R3", "Recirc Pump On - R1", "Recirc Pump On - R2", "Recirc Pump On - R3", "Recirc Pump On - R4", "Recirc Pump On - R5", "Recirc Pump On - R6", "SW_LED - Ink Valve - R4", "SW_LED - Ink Valve - R5", "SW_LED - Ink Valve - R6"] ("DOs")
                  }
                  frame "Ink Valve Switch - R1", "SW - Ink Valve - R1" {
                    (unwired) "SW_LED - Ink Valve - R1"
                    w370 = T14[] [enum."Ink Flow Valve Open - R1", enum."SW_LED - Ink Valve - R1", enum."Recirc Pump On - R1"] items=["None", "Meniscus Valve Open - R1", "Meniscus Valve Open - R2", "Meniscus Valve Open - R3", "Meniscus Valve Open - R4", "Meniscus Valve Open - R5", "Meniscus Valve Open - R6", "Ink Flow Valve Open - R1", "Ink Flow Valve Open - R2", "Ink Flow Valve Open - R3", "Ink Flow Valve Open - R4", "Ink Flow Valve Open - R5", "Ink Flow Valve Open - R6", "SW_LED - Ink Valve - R1", "SW_LED - Ink Valve - R2", "SW_LED - Ink Valve - R3", "Recirc Pump On - R1", "Recirc Pump On - R2", "Recirc Pump On - R3", "Recirc Pump On - R4", "Recirc Pump On - R5", "Recirc Pump On - R6", "SW_LED - Ink Valve - R4", "SW_LED - Ink Valve - R5", "SW_LED - Ink Valve - R6"]  # DOs
                    n104 = Format Into String(format string="%s", ICP2-DO_Channel_Names."SW_LED - Ink Valve - R1" ("DO Channel")) -> (resulting string=w366:string)  [unwired: 2 in, 1 out]
                  }
                  frame "Ink Valve Switch - R2", "SW - Ink Valve - R2" {
                    w373 = T14[] [enum."Ink Flow Valve Open - R2", enum."SW_LED - Ink Valve - R2", enum."Recirc Pump On - R2"] items=["None", "Meniscus Valve Open - R1", "Meniscus Valve Open - R2", "Meniscus Valve Open - R3", "Meniscus Valve Open - R4", "Meniscus Valve Open - R5", "Meniscus Valve Open - R6", "Ink Flow Valve Open - R1", "Ink Flow Valve Open - R2", "Ink Flow Valve Open - R3", "Ink Flow Valve Open - R4", "Ink Flow Valve Open - R5", "Ink Flow Valve Open - R6", "SW_LED - Ink Valve - R1", "SW_LED - Ink Valve - R2", "SW_LED - Ink Valve - R3", "Recirc Pump On - R1", "Recirc Pump On - R2", "Recirc Pump On - R3", "Recirc Pump On - R4", "Recirc Pump On - R5", "Recirc Pump On - R6", "SW_LED - Ink Valve - R4", "SW_LED - Ink Valve - R5", "SW_LED - Ink Valve - R6"]  # DOs
                  }
                  frame "Ink Valve Switch - R3", "SW - Ink Valve - R3" {
                    w376 = T14[] [enum."Ink Flow Valve Open - R3", enum."SW_LED - Ink Valve - R3", enum."Recirc Pump On - R3"] items=["None", "Meniscus Valve Open - R1", "Meniscus Valve Open - R2", "Meniscus Valve Open - R3", "Meniscus Valve Open - R4", "Meniscus Valve Open - R5", "Meniscus Valve Open - R6", "Ink Flow Valve Open - R1", "Ink Flow Valve Open - R2", "Ink Flow Valve Open - R3", "Ink Flow Valve Open - R4", "Ink Flow Valve Open - R5", "Ink Flow Valve Open - R6", "SW_LED - Ink Valve - R1", "SW_LED - Ink Valve - R2", "SW_LED - Ink Valve - R3", "Recirc Pump On - R1", "Recirc Pump On - R2", "Recirc Pump On - R3", "Recirc Pump On - R4", "Recirc Pump On - R5", "Recirc Pump On - R6", "SW_LED - Ink Valve - R4", "SW_LED - Ink Valve - R5", "SW_LED - Ink Valve - R6"]  # DOs
                  }
                  frame "Ink Valve Switch - R4", "SW - Ink Valve - R4" {
                    w379 = T14[] [enum."Ink Flow Valve Open - R4", enum."SW_LED - Ink Valve - R4", enum."Recirc Pump On - R4"] items=["None", "Meniscus Valve Open - R1", "Meniscus Valve Open - R2", "Meniscus Valve Open - R3", "Meniscus Valve Open - R4", "Meniscus Valve Open - R5", "Meniscus Valve Open - R6", "Ink Flow Valve Open - R1", "Ink Flow Valve Open - R2", "Ink Flow Valve Open - R3", "Ink Flow Valve Open - R4", "Ink Flow Valve Open - R5", "Ink Flow Valve Open - R6", "SW_LED - Ink Valve - R1", "SW_LED - Ink Valve - R2", "SW_LED - Ink Valve - R3", "Recirc Pump On - R1", "Recirc Pump On - R2", "Recirc Pump On - R3", "Recirc Pump On - R4", "Recirc Pump On - R5", "Recirc Pump On - R6", "SW_LED - Ink Valve - R4", "SW_LED - Ink Valve - R5", "SW_LED - Ink Valve - R6"]  # DOs
                  }
                  frame "Ink Valve Switch - R5", "SW - Ink Valve - R5" {
                    w382 = T14[] [enum."Ink Flow Valve Open - R5", enum."SW_LED - Ink Valve - R5", enum."Recirc Pump On - R5"] items=["None", "Meniscus Valve Open - R1", "Meniscus Valve Open - R2", "Meniscus Valve Open - R3", "Meniscus Valve Open - R4", "Meniscus Valve Open - R5", "Meniscus Valve Open - R6", "Ink Flow Valve Open - R1", "Ink Flow Valve Open - R2", "Ink Flow Valve Open - R3", "Ink Flow Valve Open - R4", "Ink Flow Valve Open - R5", "Ink Flow Valve Open - R6", "SW_LED - Ink Valve - R1", "SW_LED - Ink Valve - R2", "SW_LED - Ink Valve - R3", "Recirc Pump On - R1", "Recirc Pump On - R2", "Recirc Pump On - R3", "Recirc Pump On - R4", "Recirc Pump On - R5", "Recirc Pump On - R6", "SW_LED - Ink Valve - R4", "SW_LED - Ink Valve - R5", "SW_LED - Ink Valve - R6"]  # DOs
                  }
                  frame "Ink Valve Switch - R6", "SW - Ink Valve - R6" {
                    w385 = T14[] [enum."Ink Flow Valve Open - R6", enum."SW_LED - Ink Valve - R6", enum."Recirc Pump On - R6"] items=["None", "Meniscus Valve Open - R1", "Meniscus Valve Open - R2", "Meniscus Valve Open - R3", "Meniscus Valve Open - R4", "Meniscus Valve Open - R5", "Meniscus Valve Open - R6", "Ink Flow Valve Open - R1", "Ink Flow Valve Open - R2", "Ink Flow Valve Open - R3", "Ink Flow Valve Open - R4", "Ink Flow Valve Open - R5", "Ink Flow Valve Open - R6", "SW_LED - Ink Valve - R1", "SW_LED - Ink Valve - R2", "SW_LED - Ink Valve - R3", "Recirc Pump On - R1", "Recirc Pump On - R2", "Recirc Pump On - R3", "Recirc Pump On - R4", "Recirc Pump On - R5", "Recirc Pump On - R6", "SW_LED - Ink Valve - R4", "SW_LED - Ink Valve - R5", "SW_LED - Ink Valve - R6"]  # DOs
                  }
                }
                "SW LED DO" <- w316
                n105 = call "Get DAQData Dict.vi"("DAQ"=w319) -> ("DAQ Data Dict DVR"=w320:T9, "DAQ"=w318:refnum<class "DAQ.lvclass">)  [unwired: 8 in, 1 out]
                n106 = call <vilib>:"Get Dynamic CVT Data.vi"("error in (no error)"=w324, "DataName"=w316, "dCVT DVR"=w320) -> ("error out"=w322:errorcluster, "found"=w323:bool, "value"=w321:variant)  [unwired: 5 in, 1 out]
                "found" <- w323
                n107 = call "Get DAQ Boolean Data Value.vi"("DAQ"=w318, "Name"=w316) -> ("DAQ"=w317:refnum<class "DAQ.lvclass">, "Value"=→"SWLED 2":bool)  [unwired: 11 in, 1 out]
                n108 = case shown="True" w323 {
                  tunnel: w329 -> [_ w340]
                  tunnel: w328 -> [_ w339]
                  tunnel: [w330 w338] -> w327
                  tunnel: w326 -> [_ w337]
                  tunnel: w317 -> [_ w336]
                  tunnel: w322 -> [w330 w333]
                  tunnel: w321 -> [_ w335]
                  frame False {
                  }
                  frame True {
                    n109 = Variant To Data(error in=w333, type=FALSE, Variant=w335) -> (data=w331:bool, error out=w332:errorcluster)
                    "SWLED" <- w331
                    n110 = case shown="True" w331 {
                      tunnel: w336 -> [w358 w363]
                      tunnel: w332 -> [w348 w360]
                      tunnel: w340 -> [w357 w362]
                      tunnel: [w355 w359] -> w338
                      tunnel: w339 -> [w354 _]
                      tunnel: w337 -> [w341 _]
                      frame False {
                        n111 = call-dynamic "Read ProcessMode.vi"("error in (no error)"=w348, "TopLevel in"=w354) -> ("error out"=w350:errorcluster, "ProcessMode"=w351:T17, "TopLevel out"=w353:refnum<class "TopLevel.lvclass">)  [unwired: 7 in]
                        n112 = call <userlib>:"Get Strings from Enum__ogtk.vi"("error in (no error)"=w350, "Enum"=w351) -> ("error out"=w352:errorcluster, "String Value"=w349:string)  [unwired: 6 in, 2 out]
                        n113 = call "GetProcessModeParams.vi"("error in (no error)"=w352, "ModeName"=w349, "TopLevel in"=w353) -> ("error out"=w342:errorcluster, "ProcessModeValues"=w347:T18)  [unwired: 6 in, 1 out]
                        n114 = Unbundle By Name(w347) -> ("Head Enable"=w346:bool[], "Recirc[]"=w345:bool[])
                        n115 = Index Array(array=w346, index=w341) -> ()  [unwired: 1 out]
                        n116 = Index Array(array=w345, index=w341) -> (element=w343:bool)
                        n117 = Build Array (concatenate)(bool[] [TRUE, TRUE] ("Values"), w343) -> (w344:bool[])
                        n118 = call "Set DO State (automation mode) Multiple.vi"("error in (no error)"=w342, "Values"=w344, "DOs"=w357, "DAQ in"=w358) -> ("error out"=w355:errorcluster)  [unwired: 6 in, 1 out]
                      }
                      frame True {
                        n119 = call "Set DO State (automation mode) Multiple.vi"("error in (no error)"=w360, "Values"=bool[] [FALSE, FALSE, FALSE], "DOs"=w362, "DAQ in"=w363) -> ("error out"=w359:errorcluster)  [unwired: 6 in, 1 out]
                      }
                    }
                  }
                }
              }
              frame "old LED6" {
                n120 = Format Into String(format string="%s", error in=w419, ICP2-DO_Channel_Names."Ink Flow Valve Open - R6" ("DO Channel")) -> (resulting string=w427:string, error out=w422:errorcluster)  [unwired: 1 in]
                n121 = call "Generate Invert DO DAQ Out Cmd Event.vi"("mode (manual)"=TD_DAQ_Output_EventSenderMode-enum."automation", "error in (no error)"=w422, "DO IOName"=w427, "DAQ"=w426) -> ("error out"=w421:errorcluster, "DAQ"=w423:refnum<class "DAQ.lvclass">)  [unwired: 6 in]
                n122 = Format Into String(format string="%s", error in=w421, ICP2-DO_Channel_Names."SW_LED - Ink Valve - R6" ("DO Channel")) -> (resulting string=w418:string, error out=w420:errorcluster)  [unwired: 1 in]
                n123 = call "Generate Invert DO DAQ Out Cmd Event.vi"("mode (manual)"=TD_DAQ_Output_EventSenderMode-enum."automation", "error in (no error)"=w420, "DO IOName"=w418, "DAQ"=w423) -> ("error out"=w410:errorcluster, "DAQ"=w411:refnum<class "DAQ.lvclass">)  [unwired: 6 in]
                n124 = Format Into String(format string="%s", error in=w410, ICP2-DO_Channel_Names."Recirc Pump On - R6" ("DO Channel")) -> (resulting string=w413:string, error out=w412:errorcluster)  [unwired: 1 in]
                n125 = call "Generate Invert DO DAQ Out Cmd Event.vi"("mode (manual)"=TD_DAQ_Output_EventSenderMode-enum."automation", "error in (no error)"=w412, "DO IOName"=w413, "DAQ"=w411) -> ("error out"=w409:errorcluster)  [unwired: 6 in, 1 out]
              }
            }
          }
          event User Event {
            n126 = event-data() -> ()  [unwired: 1 in, 5 out]
            n127 = call <vilib>:"Add State(s) to Queue__JKI_lib_State_Machine.vi"("State(s) in Front (\"\")"="Macro: Exit" ("State(s) in Front (\"\")"), "State(s) in (\"\")"=w431) -> ("States Out"=w432:string)  [unwired: 13 in]
          }
          event User Event {
            w436 = "Macro: Exit"  # Macro: Exit
            # "This notifier needs to be fired as the last step of the exit macro sequence. This is the handshaking."
            n128 = event-data() -> ("notifier out"=w435:refnum<notifier>)  [unwired: 1 in]
            n129 = Bundle By Name(cluster=w438, "Core.process sync notifier"=w435) -> (w437:T1)
          }
          event "Stop Process": Value Change {
            n130 = event-data() -> ()  [unwired: 1 in, 1 out]
            n131 = call <vilib>:"Add State(s) to Queue__JKI_lib_State_Machine.vi"("State(s) in Front (\"\")"="Macro: Exit", "State(s) in (\"\")"=w440) -> ("States Out"=w442:string)  [unwired: 13 in]
          }
          event "inject error": Value Change {
            n132 = event-data() -> ()  [unwired: 1 in, 6 out]
          }
        }
      }
      frame "Process Sync" {
        # "#TODO AD fix this after deleting"
        # "KT 2018-0211\nuncommented DAQ thread's ThreadSync at shutdown"
        # "Rendezvous sync with DAQ\nthreads; only for startup,\nnot shutdown"
        n133 = Unbundle By Name(w457) -> ("Core.process sync notifier"=w456:refnum<notifier>, "ThreadSyncRndzv"=w452:T7)  [unwired: 1 out]
        n134 = case shown="False" FALSE {
          tunnel: w455 -> [w467 w469]
          tunnel: [w466 w469] -> w454
          tunnel: w452 -> [w465 _]
          frame False {
            # "timeout up to 1 min"
            n135 = call <vilib>:"Wait at Rendezvous.vi"("error in (no error)"=w467, "ms timeout (-1)"=60000, "rendezvous"=w465) -> ("error out"=w466:errorcluster)  [unwired: 2 in, 2 out]
          }
          frame True {
          }
        }
        n136 = call <userlib>:"Wait (ms)__ogtk.vi"("error in (no error)"=w454, "milliseconds to wait"=u32 2000) -> ("error out"=w450:errorcluster)  [unwired: 8 in, 1 out]
        n137 = disable-structure shown="Enabled" {
          disable-tunnel: w456 -> [w463 _]
          disable-tunnel: [w462 w464] -> w453
          disable-tunnel: w450 -> [w460 w464]
          frame Enabled {
            n138 = Send Notification(notification=TRUE, notifier=w463, error in (no error)=w460) -> (error out=w462:errorcluster)  [unwired: 1 out]
          }
          frame Disabled {
          }
        }
        n139 = call <vilib>:"Clear Errors.vi"("error in (no error)"=w453) -> ("error out"=w448:errorcluster)  [unwired: 5 in, 1 out]
      }
      frame "Error Handler" {
        n140 = disable-structure shown="Enabled" {
          disable-tunnel: w473 -> [w481 w483]
          disable-tunnel: w472 -> [w480 _]
          disable-tunnel: [w479 errorcluster {"status"=FALSE, "code"=0, "source"=""} ("error constant")] -> w470
          frame Enabled {
            n141 = Concatenate Strings("Previous State: ", w480) -> (w477:string)
            n142 = call "Handle Error SM.vi"("error in (no error)"=w481, "CustomMessage"=w477) -> ("error out"=w479:errorcluster)  [unwired: 7 in, 2 out]
          }
          frame Disabled {
            n143 = call <vilib>:"General Error Handler.vi"("error in (no error)"=w483) -> ()  [unwired: 10 in, 5 out]
          }
        }
        n144 = call <vilib>:"Add State(s) to Queue__JKI_lib_State_Machine.vi"("State(s) in (\"\")"=w476) -> ("States Out"=w475:string)  [unwired: 14 in]
      }
      frame "CleanUp" {
        # "Cleanup any data and references, here. (this is called automatically, by the Macro: Exit)"
        n145 = Unbundle By Name(w486) -> ("Core.Current VI Ref"=w489:refnum<vi>)
        n146 = Close Reference(reference=w489, error in (no error)=w488) -> (error out=w487:errorcluster)
      }
      frame "Exit", "Quit" {
        n147 = Unbundle By Name(w491) -> ("ThreadSyncRndzv"=w490:T7)
        n148 = flat-sequence {
          tunnel: w490 -> [w496]
          frame #0 {
            n149 = call <vilib>:"Destroy Rendezvous.vi"("rendezvous"=w496) -> ()  [unwired: 5 in, 2 out]
          }
        }
      }
      frame "------ Data ------" {
      }
      frame "Data: Initialize" {
        n150 = control-ref of="Current VI Reference"() -> (w507:refnum<vi>)
        n151 = Bundle By Name(cluster=w502, "Core.Current VI Ref"=w507, "Core.process sync notifier"="start process sync notifier", "quitting"=FALSE, "Timer.Expired"=TRUE) -> (w505:T1)
      }
      frame "------ Macro ------" {
      }
      frame "Macro: Initialize" {
        # "Initialization Macro (This is called once, when the VI starts)"
        n152 = call <vilib>:"Add State(s) to Queue__JKI_lib_State_Machine.vi"("State(s) in Front (\"\")"=w514, "State(s) in (\"\")"=w519) -> ("States Out"=w518:string)  [unwired: 13 in]
      }
      frame "Macro: Exit" {
        n153 = Unbundle By Name(w523) -> ("AsyncSMQ"=w522:refnum<queue>)
        n154 = Bundle By Name(cluster=w523, "quitting"=TRUE) -> (w527:T1)
        n155 = call <vilib>:"Add State to Queue with vData.vi"("queue in"=w522, "state in"="Macro: Exit", "error in"=w520) -> ("error out"=w521:errorcluster)  [unwired: 9 in, 3 out]
        n156 = call <vilib>:"Add State(s) to Queue__JKI_lib_State_Machine.vi"("State(s) in Front (\"\")"=w525, "State(s) in (\"\")"=w530) -> ("States Out"=w529:string)  [unwired: 13 in]
      }
      frame "------ UI ------" {
      }
      frame "UI: Front Panel State" {
        # "Argument"
        n157 = Unbundle By Name(w538) -> ("Core.Current VI Ref"=w539:refnum<vi>)
        n158 = case shown="\"Open\", Default" w535 {
          tunnel: w536 -> [w545 w558]
          tunnel: [w547 w559] -> w537
          tunnel: w539 -> [w546 w556]
          frame "Open", Default {
            n159 = property class="VI"(reference=w546, error in=w545) -> (reference out=w543:refnum<vi>, error out=w544:errorcluster, "Front Panel.Open"=w542:bool)
            n160 = case shown="False" w542 {
              tunnel: [w550 w553] -> w547
              tunnel: w544 -> [w549 w553]
              tunnel: w543 -> [w548 _]
              frame False {
                n161 = invoke class="VI" method="FP.Open"(reference=w548, error in=w549, "Activate"=TRUE, "State"=T15."Standard") -> (error out=w550:errorcluster)  [unwired: 1 in, 4 out]
              }
              frame True {
              }
            }
          }
          frame "Close" {
            n162 = property class="VI"(reference=w556, error in=w558) -> (reference out=w555:refnum<vi>, error out=w557:errorcluster, "Front Panel.Open"=w554:bool)
            n163 = case shown="True" w554 {
              tunnel: [w560 w563] -> w559
              tunnel: w557 -> [w560 w562]
              tunnel: w555 -> [_ w561]
              frame False {
              }
              frame True {
                n164 = invoke class="VI" method="FP.Close"(reference=w561, error in=w562) -> (error out=w563:errorcluster)  [unwired: 1 in, 2 out]
              }
            }
          }
        }
      }
      frame "UI: Register Events" {
        n165 = Unbundle By Name(w573) -> ("Self Reference"=w570:refnum<class "DAQ.lvclass">, "TopLevel"=w564:refnum<class "TopLevel.lvclass">)
        n166 = call-dynamic "GetEvents_TopLevel.vi"("error in (no error)"=w565, "TopLevel in"=w564) -> ("error out"=w566:errorcluster, "UserEvents"=w568:T19)  [unwired: 7 in, 1 out]
        n167 = call "Get Public Events.vi"("error in (no error)"=w566, "DAQ"=w570) -> ("error out"=w569:errorcluster, "PublicEvents"=w571:T20)  [unwired: 7 in, 1 out]
        n168 = Unbundle By Name(w568) -> ("Exit Event"=w567:refnum<user-event>)
        n169 = register-events(error in=w569, w571, w567) -> (reference out=w574:refnum<event-registration>, error out=w572:errorcluster)  [unwired: 1 in]
      }
      frame "UI: Unregister Events" {
        n170 = Unregister For Events(event registration refnum=w577, error in=w576) -> (error out=w578:errorcluster)
        n171 = call <vilib>:"Clear Errors.vi"("error in (no error)"=w578) -> ()  [unwired: 5 in, 2 out]
      }
      frame "------ Action ------" {
      }
      frame "Action: SendPurgeAck" {
        n172 = Unbundle By Name(w589) -> ("TopLevel"=w587:refnum<class "TopLevel.lvclass">)
        n173 = call-dynamic "Generate PurgeRequestEvent.vi"("error in (no error)"=w585, "Command"="Done" ("CmdMsg"), "TopLevel in"=w587) -> ("error out"=w586:errorcluster)  [unwired: 7 in, 1 out]
      }
      frame "Action: Request Purge" {
        # "Launch async here"
        n174 = Unbundle By Name(w607) -> ("TopLevel"=w597:refnum<class "TopLevel.lvclass">)
        n175 = vi-ref "TopLevel.lvclass:PurgeRequestWindow--Process.vi"() -> (w606:refnum<vi>)
        n176 = property class="VI (strict)"(reference=w606, error in=w596) -> (reference out=w604:refnum<vi>, error out=w599:errorcluster, "Path"=w605:path)
        n177 = Open VI Reference(type specifier VI Refnum (for type only)=w604, vi path=w605, options=128, error in (no error)=w599) -> (vi reference=w602:refnum<vi>, error out=w600:errorcluster)  [unwired: 2 in]
        n178 = call-by-ref "Start Asynchronous Call"(reference=w602, error in=w600, "TopLevel In"=w597) -> (reference out=w598:refnum<vi>, error out=w601:errorcluster)  [unwired: 11 in]
        n179 = Bundle By Name(cluster=w607, "Timer.Expired"=FALSE) -> (w593:T1)
        n180 = Close Reference(reference=w598, error in (no error)=w601) -> (error out=w595:errorcluster)
        n181 = call <vilib>:"Clear Errors.vi"("error in (no error)"=w595) -> ("error out"=w594:errorcluster)  [unwired: 5 in, 1 out]
      }
      frame "Action: Timer" {
        n182 = case shown="\"Init\"" w612 {
          tunnel: w610 -> [w616 w621 w624 w627 w631]
          tunnel: [w616 w620 w623 w626 w630] -> w611
          frame "False", Default {
          }
          frame "Enable" {
            n183 = Get Date/Time In Seconds() -> (seconds since 1Jan1904=w618:timestamp)
            n184 = Bundle By Name(cluster=w621, "Timer.Enable"=TRUE, "Timer.StartTime"=w618, "Timer.Expired"=FALSE) -> (w620:T1)
          }
          frame "Disable" {
            n185 = Bundle By Name(cluster=w624, "Timer.Enable"=FALSE) -> (w623:T1)
          }
          frame "Reset" {
            n186 = Get Date/Time In Seconds() -> (seconds since 1Jan1904=w625:timestamp)
            n187 = Bundle By Name(cluster=w627, "Timer.StartTime"=w625) -> (w626:T1)
          }
          frame "Init" {
            # "not used"
            n188 = Bundle By Name(cluster=w631, "Timer.Expired"=TRUE, "Timer.Enable"=TRUE) -> (w630:T1)
          }
        }
      }
    }
  }
  n189 = Merge Errors(w6, w7) -> (→"error out":errorcluster)
